vi "filefolderTESTING.vi"() -> ()   [LabVIEW 2020]
panel:
  in  "Weight":enum16{"0g", "300g", "600g", "900g"}(ring)
  in  "Test Type":enum16{"Static", "Dynamic"}(ring)
  in  "Group ID":enum16{"G1", "G2"}(ring)
  in  "Patient ID":string caption="Participant Name (FirstLast)"
  in  "Path":path=path "C:/Users/rsKite/Documents/FSR DATA"
  in  "Trial (Round)":string caption="Participant Name (FirstLast)"
  out "File Name":string
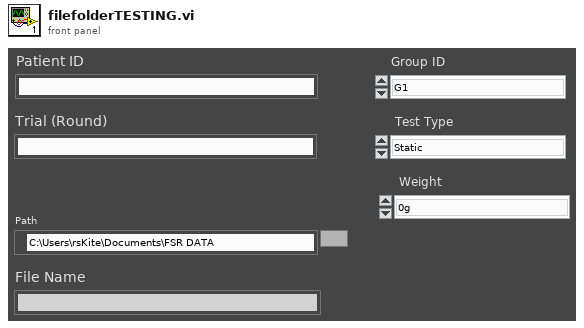
[diagram p1: front panel]
types:
  T1 = enum16{"open", "replace", "create", "open or create", "replace or create", "replace or create with confirmation"}
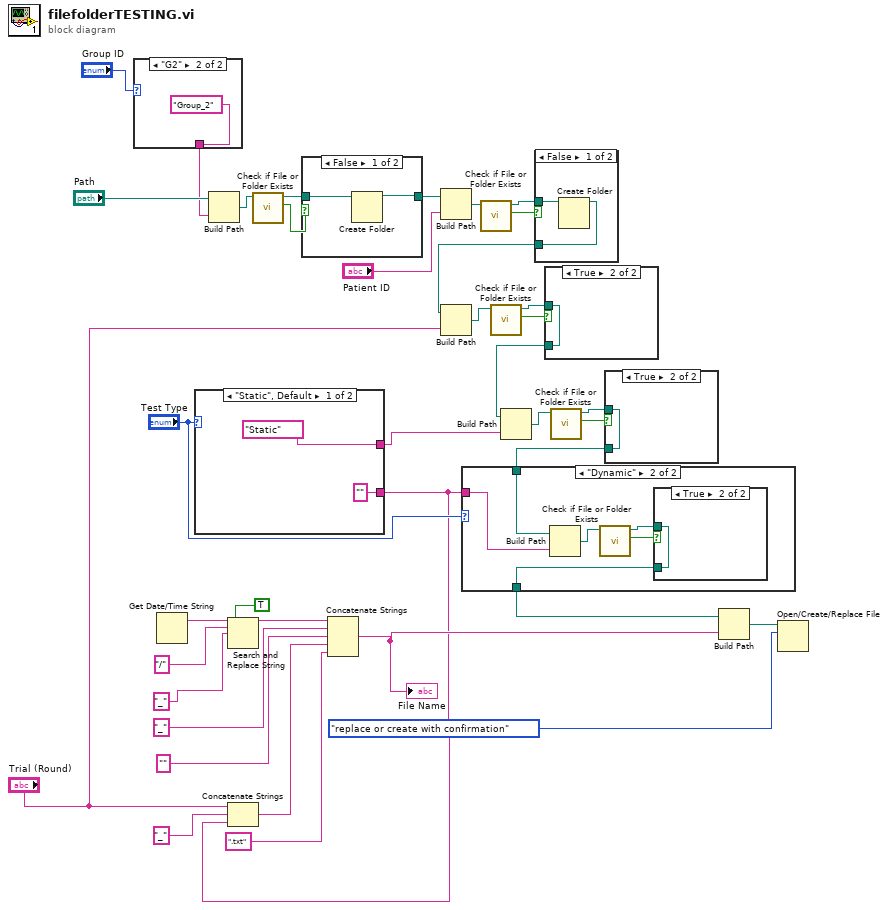
[diagram p0: block diagram]
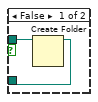
[diagram p3: hidden frame]
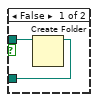
[diagram p4: hidden frame]
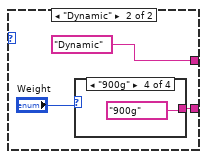
[diagram p5: hidden frame]
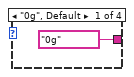
[diagram p6: hidden frame]
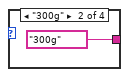
[diagram p7: hidden frame]
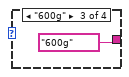
[diagram p8: hidden frame]
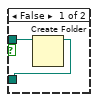
[diagram p9: hidden frame]
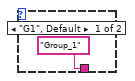
[diagram p11: hidden frame]
diagram:
  n1 = case shown="\"G2\"" "Group ID" {
    tunnel: ["Group_1" "Group_2"] -> w20
    frame "G1", Default {
    }
    frame "G2" {
    }
  }
  n2 = Get Date/Time String() -> (date string=w38:string)  [unwired: 3 in, 1 out]
  n3 = case shown="\"Static\", Default" "Test Type" {
    tunnel: ["Static" "Dynamic"] -> w5
    tunnel: ["" w43] -> w1
    frame "Static", Default {
    }
    frame "Dynamic" {
      n4 = case shown="\"900g\"" "Weight" {
        tunnel: ["0g" "300g" "600g" "900g"] -> w43
        frame "0g", Default {
        }
        frame "300g" {
        }
        frame "600g" {
        }
        frame "900g" {
        }
      }
    }
  }
  n5 = Build Path(base path="Path", name or relative path=w20) -> (appended path=w24:path)
  n6 = Search and Replace String(replace all?=TRUE ("replace all? (F)"), input string=w38, search string="/", replace string="_" ("replace string (\"\")")) -> (result string=w36:string)  [unwired: 4 in, 3 out]
  n7 = Concatenate Strings("Trial (Round)", "_" ("string"), w1) -> (w37:string)
  n8 = call <vilib>:"Check if File or Folder Exists.vi"("path"=w24) -> ("file or folder exists?"=w23:bool, "dup path"=w22:path)  [unwired: 8 in, 1 out]
  n9 = case shown="False" w23 {
    tunnel: w22 -> [w51 w52]
    tunnel: [w50 w52] -> w19
    frame False {
      n10 = Create Folder(path (use dialog)=w51) -> (created path=w50:path)  [unwired: 2 in, 2 out]
    }
    frame True {
    }
  }
  n11 = Concatenate Strings(w36, "_" ("string"), "" ("string"), w37, ".txt" ("string")) -> (w35:string)
  "File Name" <- w35
  n12 = Build Path(base path=w19, name or relative path="Patient ID") -> (appended path=w18:path)
  n13 = call <vilib>:"Check if File or Folder Exists.vi"("path"=w18) -> ("file or folder exists?"=w17:bool, "dup path"=w16:path)  [unwired: 8 in, 1 out]
  n14 = case shown="False" w17 {
    tunnel: w16 -> [w54 w55]
    tunnel: [w53 w55] -> w11
    frame False {
      n15 = Create Folder(path (use dialog)=w54) -> (created path=w53:path)  [unwired: 2 in, 2 out]
    }
    frame True {
    }
  }
  n16 = Build Path(base path=w11, name or relative path="Trial (Round)") -> (appended path=w12:path)
  n17 = call <vilib>:"Check if File or Folder Exists.vi"("path"=w12) -> ("file or folder exists?"=w13:bool, "dup path"=w14:path)  [unwired: 8 in, 1 out]
  n18 = case shown="True" w13 {
    tunnel: w14 -> [w57 w58]
    tunnel: [w56 w58] -> w6
    frame False {
      n19 = Create Folder(path (use dialog)=w57) -> (created path=w56:path)  [unwired: 2 in, 2 out]
    }
    frame True {
    }
  }
  n20 = Build Path(base path=w6, name or relative path=w5) -> (appended path=w10:path)
  n21 = call <vilib>:"Check if File or Folder Exists.vi"("path"=w10) -> ("file or folder exists?"=w9:bool, "dup path"=w8:path)  [unwired: 8 in, 1 out]
  n22 = case shown="True" w9 {
    tunnel: w8 -> [w60 w61]
    tunnel: [w59 w61] -> w3
    frame False {
      n23 = Create Folder(path (use dialog)=w60) -> (created path=w59:path)  [unwired: 2 in, 2 out]
    }
    frame True {
    }
  }
  n24 = case shown="\"Dynamic\"" "Test Type" {
    tunnel: w3 -> [w62 w65]
    tunnel: w1 -> [_ w64]
    tunnel: [w62 w63] -> w2
    frame "Static", Default {
    }
    frame "Dynamic" {
      n25 = Build Path(base path=w65, name or relative path=w64) -> (appended path=w66:path)
      n26 = call <vilib>:"Check if File or Folder Exists.vi"("path"=w66) -> ("file or folder exists?"=w67:bool, "dup path"=w68:path)  [unwired: 8 in, 1 out]
      n27 = case shown="True" w67 {
        tunnel: w68 -> [w70 w71]
        tunnel: [w69 w71] -> w63
        frame False {
          n28 = Create Folder(path (use dialog)=w70) -> (created path=w69:path)  [unwired: 2 in, 2 out]
        }
        frame True {
        }
      }
    }
  }
  n29 = Build Path(base path=w2, name or relative path=w35) -> (appended path=w28:path)
  n30 = Open/Create/Replace File(file path (use dialog)=w28, operation (0:open)=T1."replace or create with confirmation") -> ()  [unwired: 4 in, 3 out]
